vi "Test Compare Numerical Values Outside Tolerance Fails.vi"(8 "error in (no error)":errorcluster, 11 "Test Case In":refnum<class "Tolerant Numeric Comparator Test.lvclass">) -> (0 "error out":errorcluster, 3 "Test Case Out":refnum<class "Tolerant Numeric Comparator Test.lvclass">)   [LabVIEW 2020, in "Tolerant Numeric Comparator Test.lvclass"]
uses:
  Tolerant Numeric Comparator Test.lvclass
  C:/Program Files (x86)/National Instruments/LabVIEW 2020/vi.lib/Astemes/LUnit/Test Case.lvclass
  <vilib>/Astemes/LUnit/Test Case.lvclass/Test Case.ctl
  <vilib>/Astemes/LUnit/Append Pass Result.vi
  <vilib>/Astemes/LUnit/Append Fail Result.vi
  Mock VI Call/Mock VI Call.lvclass
  C:/git/astemes-lmock/sandbox/Call/VI Call.lvclass
  Tolerant Numeric Comparator/Tolerant Numeric Comparator.lvclass
  <vilib>/Astemes/LUnit/Test Case.lvclass
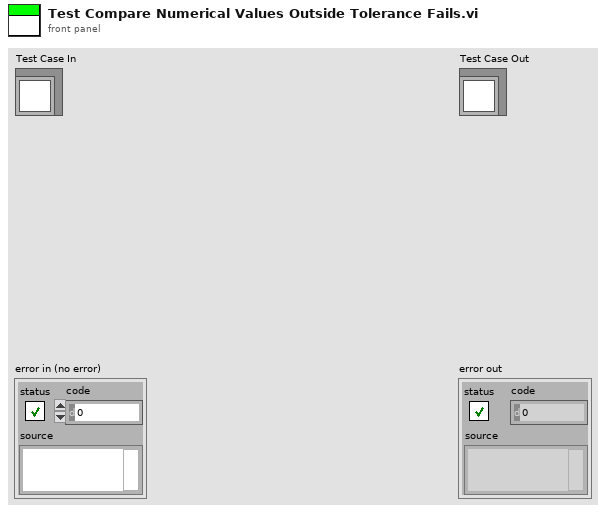
[diagram p1: front panel]
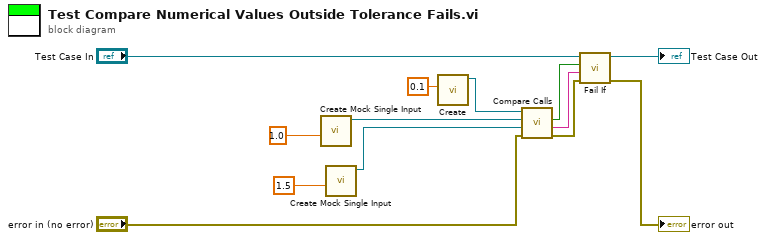
[diagram p0: block diagram]
diagram:
  n1 = call "Create Mock Single Input.vi"("Control value"=1.0) -> ("Mock VI Call Out"=w11:refnum<class "Mock VI Call.lvclass">)  [unwired: 9 in, 1 out]
  n2 = call "Create Mock Single Input.vi"("Control value"=1.5) -> ("Mock VI Call Out"=w10:refnum<class "Mock VI Call.lvclass">)  [unwired: 9 in, 1 out]
  n3 = call "Create.vi"("Tolerance"=0.1) -> ("Tolerant Numeric Comparator"=w8:refnum<class "Tolerant Numeric Comparator.lvclass">)  [unwired: 9 in, 1 out]
  n4 = call-dynamic "Compare Calls.vi"("error in (no error)"="error in (no error)", "VI Call 2"=w10, "VI Call 1"=w11, "Tolerant Numeric Comparator In"=w8) -> ("error out"=w4:errorcluster, "Description"=w1:string, "Equal?"=w2:bool)  [unwired: 5 in]
  n5 = call <vilib>:"Fail If.vi"("error in (no error)"=w4, "Message"=w1, "Fail?"=w2, "LUnit Test Case In"="Test Case In") -> ("error out"=→"error out":errorcluster, "LUnit Test Case Out"=→"Test Case Out":refnum<class "Tolerant Numeric Comparator Test.lvclass">)  [unwired: 6 in]
